vi "Log Data TDMS.vi"(7 "Commnad":T1, 8 "error in (no error)":errorcluster, 10 "data":waveform(dbl)[](array[waveform]), 11 "Channel name":string[](array[string])) -> (0 "error out":errorcluster)   [LabVIEW 2016, in "User Interface.lvlib"]
uses:
  User Interface.lvlib
  Log Data Command.ctl
  Create Path Command.ctl
panel:
  in  "Time Stamp":timestamp
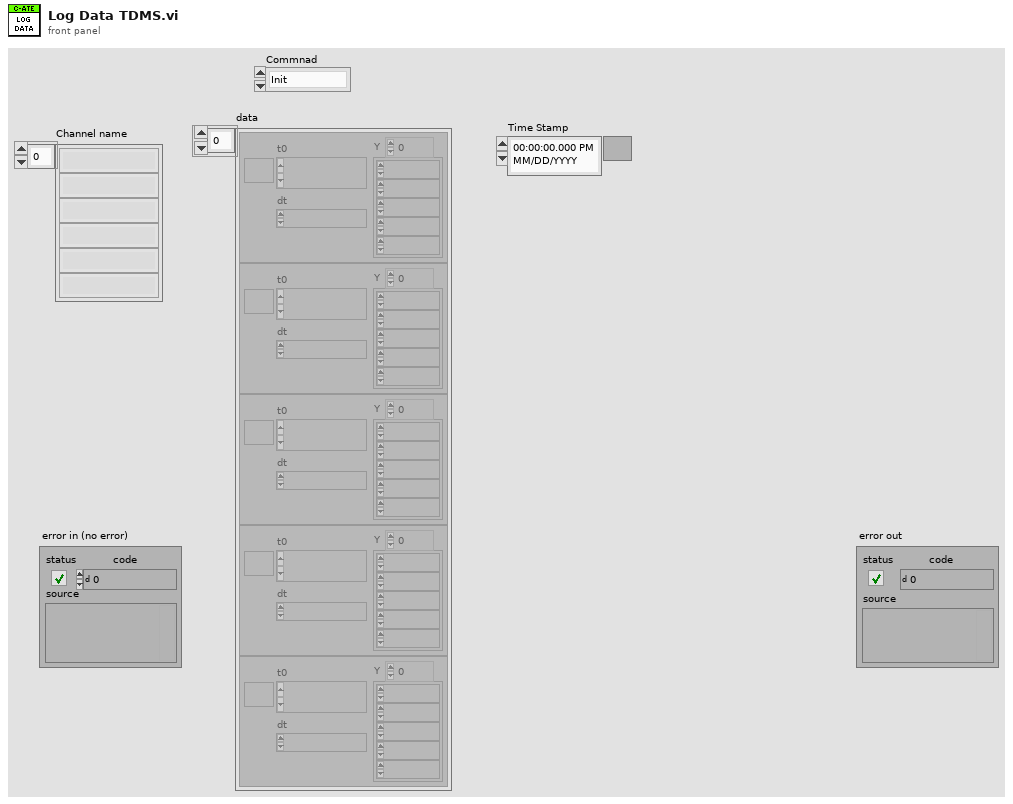
[diagram p1: front panel]
types:
  T1 = typedef "User Interface.lvlib/Log Data Command.ctl" = enum16{"Init", "Read", "Write", "Close"}
  T2 = typedef "User Interface.lvlib/Create Path Command.ctl" = enum16{"Authentication", "Hardware", "Instrument", "Data", "Action log", "Error Log"}
  T3 = enum16{"open", "open or create", "create or replace", "create", "open (read-only)"}
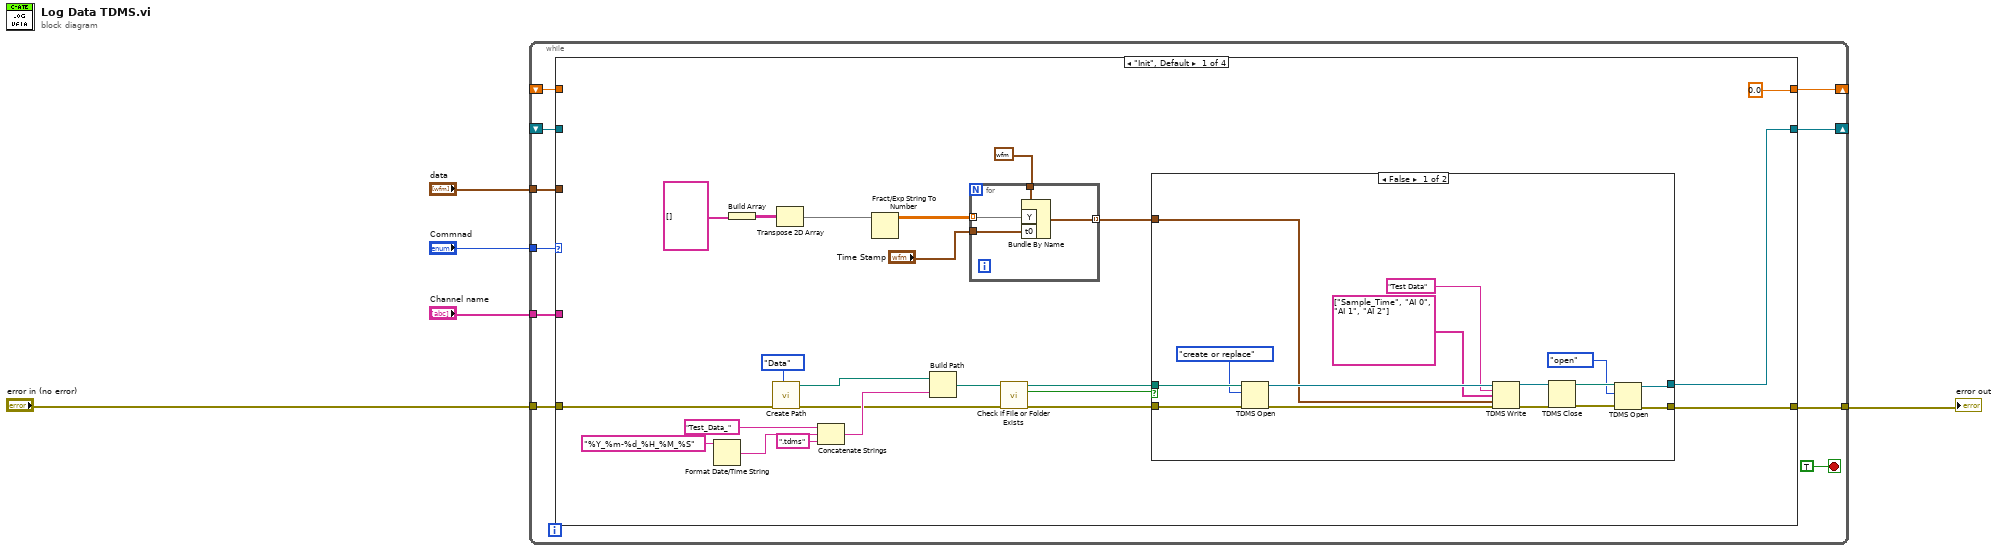
[diagram p0: block diagram]
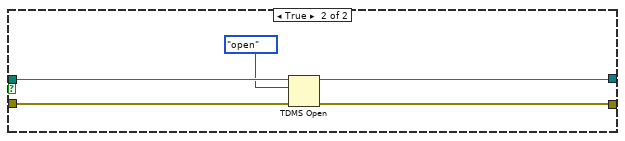
[diagram p2: hidden frame]
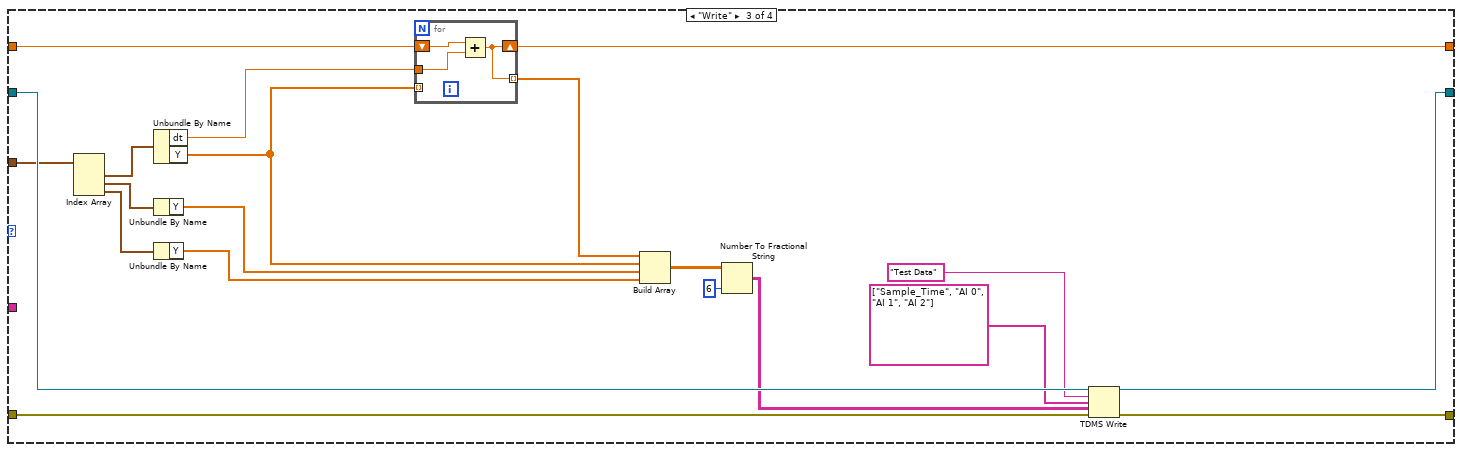
[diagram p4: hidden frame]
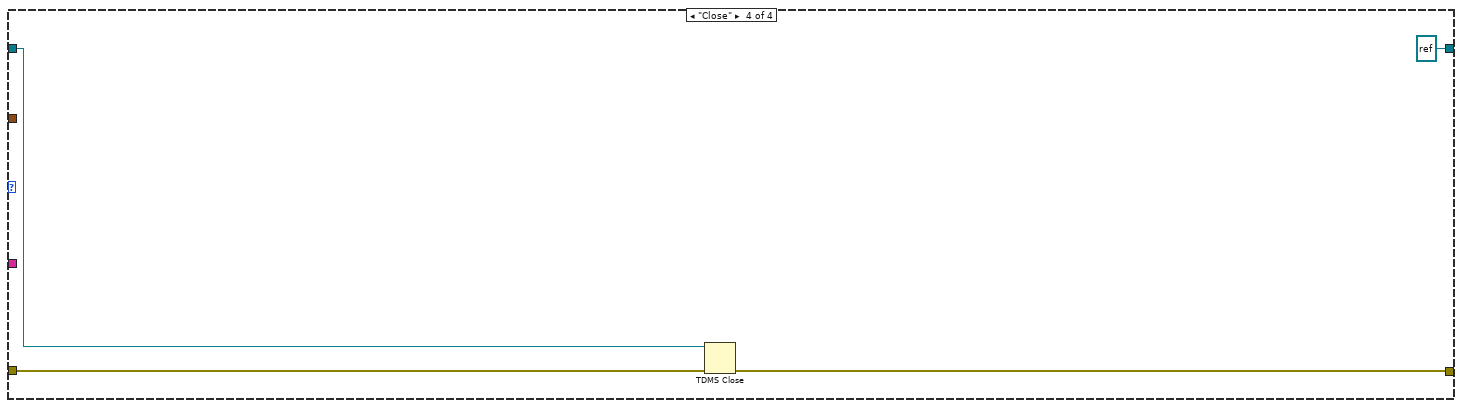
[diagram p5: hidden frame]
diagram:
  n1 = while {
    tunnel: "error in (no error)" -> [w14]
    tunnel: "Commnad" -> [w13]
    tunnel: [w12] -> w3
    shift-right: [w11] -> _
    shift-left: _ -> [w10]
    tunnel: "Channel name" -> [w9]
    tunnel: "data" -> [w8]
    shift-right: [w6] -> _
    shift-left: _ -> [w7]
    stop <- TRUE stop-if-true
    n2 = case shown="\"Init\", Default" w13 {
      tunnel: w14 -> [w38 _ w83 w90]
      tunnel: [w25 _ w80 w89] -> w12
      tunnel: [w24 w63 w81 refnum<k34> refnum ("tdms file out")] -> w11
      tunnel: w10 -> [_ w63 w82 w88]
      tunnel: w9 -> [_ _ _ _]
      tunnel: w8 -> [_ _ w74 _]
      tunnel: w7 -> [_ _ w72 _]
      tunnel: [0.0 _ w69 _] -> w6
      frame "Init", Default {
        n3 = Format Date/Time String(time format string (%c)="%Y_%m-%d_%H_%M_%S") -> (date/time string=w30:string)  [unwired: 2 in]
        n4 = Build Array(string[] []) -> (w20:string[][])
        n5 = call "Create Path.vi"("Path Command"=Create_Path_Command."Data", "error in (no error)"=w38) -> ("error out"=w26:errorcluster, "created path"=w32:path)  [unwired: 8 in]
        n6 = Transpose 2D Array(2D array=w20) -> (transposed array=w19:string[][])
        n7 = Concatenate Strings("Test_Data_" ("string"), w30, ".tdms" ("string")) -> (w28:string)
        n8 = Fract/Exp String To Number(string=w19) -> (number=w16:dbl[][])  [unwired: 3 in, 1 out]
        n9 = Build Path(base path=w32, name or relative path=w28) -> (appended path=w27:path)
        n10 = for {
          tunnel: waveform(dbl) {"t0"=timestamp(0 s since 1904-01-01), "dt"=1.0, "Y"=[]} ("waveform") -> [w42]
          tunnel: w16 -> [w41] mode=indexing
          tunnel: "Time Stamp" -> [w40]
          tunnel: [w39] -> w17 mode=indexing
          n11 = Bundle By Name(cluster=w42, "Y"=w41, "t0"=w40) -> (w39:waveform(dbl))
        }
        n12 = call <vilib>:"Check if File or Folder Exists.vi"("error in (no error)"=w26, "path"=w27) -> ("error out"=w36:errorcluster, "file or folder exists?"=w35:bool, "dup path"=w34:path)  [unwired: 7 in]
        n13 = case shown="False" w35 {
          tunnel: w36 -> [w56 w62]
          tunnel: w34 -> [w57 w61]
          tunnel: [w47 w59] -> w25
          tunnel: [w48 w60] -> w24
          tunnel: w17 -> [w46 _]
          frame False {
            n14 = TDMS Open(8:w56, 10:T3."create or replace" ("operation (0:open)"), 11:w57) -> (0:w54:errorcluster, 3:w53:refnum<k34>)  [unwired: 4 in]
            n15 = TDMS Write(0:w53, 5:"Test Data", 7:string[] ["Sample_Time", "AI 0", "AI 1", "AI 2"], 9:w46, 11:w54) -> (4:w52:refnum<k34>, 15:w51:errorcluster)  [unwired: 1 in, 2 out]
            n16 = TDMS Close(8:w51, 11:w52) -> (0:w49:errorcluster, 3:w50:path)
            n17 = TDMS Open(8:w49, 10:T3."open" ("operation (0:open)"), 11:w50) -> (0:w47:errorcluster, 3:w48:refnum<k34>)  [unwired: 4 in]
          }
          frame True {
            n18 = TDMS Open(8:w62, 10:T3."open" ("operation (0:open)"), 11:w61) -> (0:w59:errorcluster, 3:w60:refnum<k34>)  [unwired: 4 in]
          }
        }
      }
      frame "Read" {
      }
      frame "Write" {
        n19 = Index Array(array=w74) -> (element #1=w79:waveform(dbl), element #2=w78:waveform(dbl), element #3=w77:waveform(dbl))  [unwired: 3 in]
        n20 = Unbundle By Name(w79) -> ("dt"=w70:dbl, "Y"=w71:dbl[])
        n21 = Unbundle By Name(w78) -> ("Y"=w76:dbl[])
        n22 = Unbundle By Name(w77) -> ("Y"=w75:dbl[])
        n23 = for {
          shift-right: [w84] -> w69
          shift-left: w72 -> [w86]
          tunnel: w71 -> [_] mode=indexing
          tunnel: w70 -> [w85]
          tunnel: [w84] -> w68 mode=indexing
          n24 = Add(x=w86, y=w85) -> (x+y=w84:dbl)
        }
        n25 = Build Array(w68, w71, w76, w75) -> (w66:dbl[][])
        n26 = Number To Fractional String(number=w66, precision (6)=i16 6) -> (F-format string=w65:string[][])  [unwired: 2 in]
        n27 = TDMS Write(0:w82, 5:"Test Data", 7:string[] ["Sample_Time", "AI 0", "AI 1", "AI 2"], 9:w65, 11:w83) -> (4:w81:refnum<k34>, 15:w80:errorcluster)  [unwired: 1 in, 2 out]
      }
      frame "Close" {
        n28 = TDMS Close(8:w90, 11:w88) -> (0:w89:errorcluster)  [unwired: 1 out]
      }
    }
  }
  "error out" <- w3
